vi "PH_Histogram.vi"(0 "Data In":u32[](array[numeric])) -> (4 "Histogram":i32[](array[numeric]))   [LabVIEW 2009]
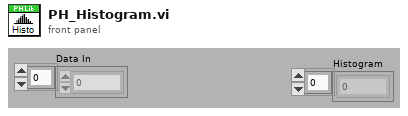
[diagram p1: front panel]
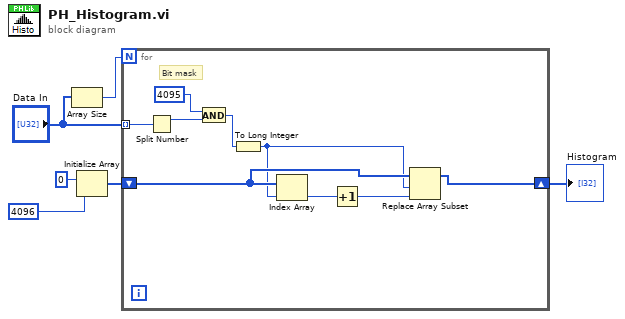
[diagram p0: block diagram]
diagram:
  n1 = Array Size(array="Data In") -> (size(s)=w1:i32)
  n2 = Initialize Array(0 ("element"), 4096 ("dimension size")) -> (w4:i32[])
  n3 = for {
    N: w1 -> [_]
    tunnel: "Data In" -> [w15] mode=indexing
    shift-right: [w7] -> w3
    shift-left: w4 -> [w10]
    # "Bit mask"
    n4 = Split Number(x=w15) -> (hi(x)=w14:u16)  [unwired: 1 out]
    n5 = And(x=u16 4095, y=w14) -> (x .and. y?=w12:u16)
    n6 = To Long Integer(number=w12) -> (32bit integer=w9:i32)
    n7 = Index Array(array=w10, index=w9) -> (element=w11:i32)
    n8 = Increment(x=w11) -> (x+1=w8:i32)
    n9 = Replace Array Subset(array=w10, new element=w8, index=w9) -> (w7:i32[])
  }
  "Histogram" <- w3
